vi "Inicio.vi"(11 "error in":errorcluster) -> (4 "Cluster":T1, 13 "notifier out":refnum<notifier>, 15 "error out":errorcluster)   [LabVIEW 2015]
uses:
  EnumEstado.ctl
  Application/ClusterM1.ctl
  Application/ClusterM2.ctl
  Application/Enum_File.ctl
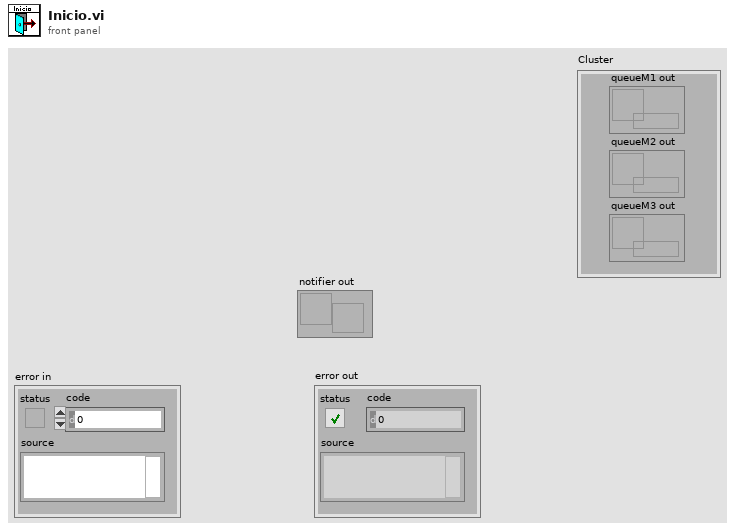
[diagram p1: front panel]
types:
  T1 = cluster{"queueM1 out":refnum<queue>, "queueM2 out":refnum<queue>, "queueM3 out":refnum<queue>}
  T2 = typedef "ClusterM2.ctl" = cluster{"timeStamp":timestamp, "Data":dbl[], "group":string}
  T3 = typedef "Enum_File.ctl" = enum16{"GET", "SET"}
  T4 = typedef "ClusterM1.ctl" = cluster{"group":string, "timeStamp":timestamp, "Temperature Ambient":dbl, "radiation":dbl, "RH":dbl, "Temperature Panel":dbl}
  T5 = enum16{"open", "open or create", "create or replace", "create", "open (read-only)"}
  T6 = typedef "EnumEstado.ctl" = enum16{"Stop", "Iniciado", "Log In", "Log Out", "Escribir", "Leer Radiacion", "Leer Temp", "Leer Humed Relat", "Leer Temp del Panel", "Leer Pot Panel", "Leer Pot Fase R", "Leer Pot Fase  S", "Leer PotFase T", "Leer Nivel Bat", "Leer Pot Generador"}
  T7 = cluster{"tdms file out":refnum<k34>, "tdms file out":refnum<k34>, "tdms file out":refnum<k34>}
  T8 = cluster{"queue out":refnum<queue>, "queue out":refnum<queue>, "queue out":refnum<queue>}
  T9 = typedef "Semaphore RefNum" = refnum<k1>
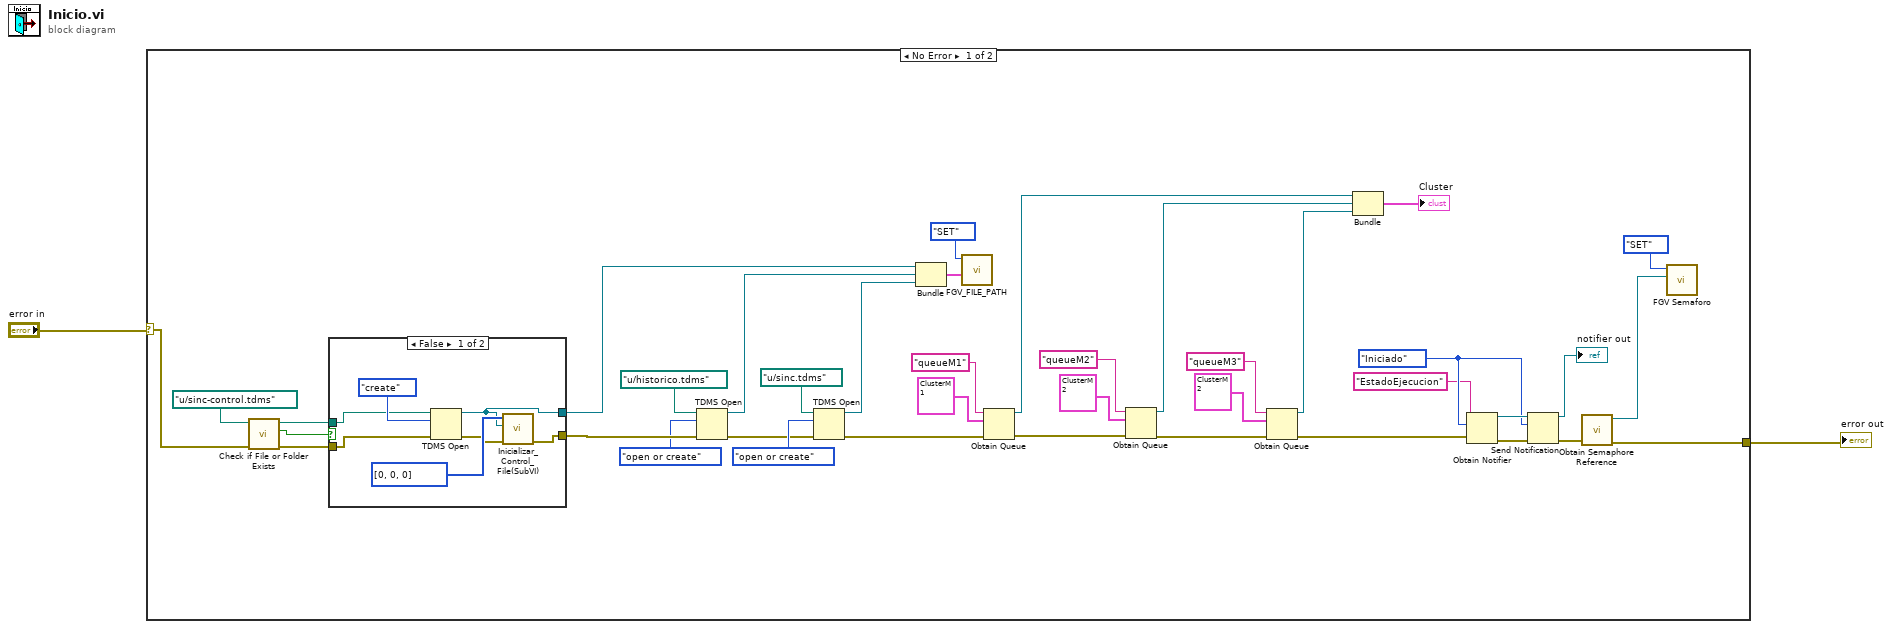
[diagram p0: block diagram]
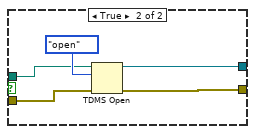
[diagram p2: hidden frame]
diagram:
  n1 = case shown="No Error" "error in" {
    selector: "error in" -> [w3 w54]
    tunnel: [w8 w54] -> w2
    frame No Error {
      w33 = EnumEstado."Iniciado"
      n2 = call <vilib>:"Check if File or Folder Exists.vi"("error in (no error)"=w3, "path"=path "u:/sinc-control.tdms" ("file path")) -> ("error out"=w6:errorcluster, "file or folder exists?"=w5:bool, "dup path"=w4:path)  [unwired: 7 in]
      n3 = case shown="False" w5 {
        tunnel: [w44 w52] -> w20
        tunnel: [w45 w51] -> w40
        tunnel: w6 -> [w42 w50]
        tunnel: w4 -> [w43 w49]
        frame False {
          n4 = TDMS Open(8:w42, 10:T5."create" ("operation (0:open)"), 11:w43) -> (0:w46:errorcluster, 3:w44:refnum<k34>)  [unwired: 4 in]
          n5 = call "Inicializar_Control_File(SubVI).vi"("error in"=w46, "tdms file"=w44, "Offsets"=i64[] [0, 0, 0]) -> ("error out"=w45:errorcluster)  [unwired: 8 in]
        }
        frame True {
          n6 = TDMS Open(8:w50, 10:T5."open" ("operation (0:open)"), 11:w49) -> (0:w51:errorcluster, 3:w52:refnum<k34>)  [unwired: 4 in]
        }
      }
      n7 = TDMS Open(8:w40, 10:T5."open or create" ("operation (0:open)"), 11:path "u:/historico.tdms" ("file path")) -> (0:w36:errorcluster, 3:w19:refnum<k34>)  [unwired: 4 in]
      n8 = TDMS Open(8:w36, 10:T5."open or create" ("operation (0:open)"), 11:path "u:/sinc.tdms" ("file path")) -> (0:w27:errorcluster, 3:w18:refnum<k34>)  [unwired: 4 in]
      n9 = Bundle("tdms file out"=w20, "tdms file out"=w19, "tdms file out"=w18) -> (w16:T7)  [unwired: 1 in]
      n10 = call "FGV_FILE_PATH.vi"("Data In"=w16, "Function"=Enum_File."SET") -> ()  [unwired: 9 in, 1 out]
      n11 = Obtain Queue(name (unnamed)="queueM1", element data type=T4 {"group"="", "timeStamp"=timestamp(0 s since 1904-01-01), "Temperature Ambient"=0.0, "radiation"=0.0, "RH"=0.0, "Temperature Panel"=0.0} ("M1"), error in (no error)=w27) -> (queue out=w12:refnum<queue>, error out=w24:errorcluster)  [unwired: 2 in, 1 out]
      n12 = Obtain Queue(name (unnamed)="queueM2", element data type=T2 {"timeStamp"=timestamp(0 s since 1904-01-01), "Data"=[], "group"=""} ("M2"), error in (no error)=w24) -> (queue out=w11:refnum<queue>, error out=w21:errorcluster)  [unwired: 2 in, 1 out]
      n13 = Obtain Queue(name (unnamed)="queueM3", element data type=T2 {"timeStamp"=timestamp(0 s since 1904-01-01), "Data"=[], "group"=""} ("M2"), error in (no error)=w21) -> (queue out=w10:refnum<queue>, error out=w15:errorcluster)  [unwired: 2 in, 1 out]
      n14 = Bundle("queue out"=w12, "queue out"=w11, "queue out"=w10) -> (→"Cluster":T8)  [unwired: 1 in]
      n15 = Obtain Notifier(name (unnamed)="EstadoEjecucion", notification data type=w33, error in (no error)=w15) -> (notifier out=w34:refnum<notifier>, error out=w35:errorcluster)  [unwired: 1 in, 1 out]
      n16 = Send Notification(notification=w33, notifier=w34, error in (no error)=w35) -> (notifier out=→"notifier out":refnum<notifier>, error out=w31:errorcluster)
      n17 = call <vilib>:"Obtain Semaphore Reference.vi"("error in (no error)"=w31) -> ("error out"=w8:errorcluster, "semaphore"=w13:T9)  [unwired: 4 in, 1 out]
      n18 = call "FGV Semaforo.vi"("semaphore"=w13, "Function"=enum16{"GET", "SET"}."SET") -> ()  [unwired: 9 in, 1 out]
    }
    frame Error {
    }
  }
  "error out" <- w2
